vi "connection state machine.vi"(11 "connection in":refnum<class "connection maintainer.lvclass">) -> ()   [LabVIEW 2015, in "connection maintainer.lvclass"]
uses:
  connection maintainer.lvclass
  communicator/communicator.lvclass/communicator.ctl
  message/communicator message.lvclass/communicator message.ctl
  connection maintainer.lvclass/connection maintainer.ctl
  message/create message.vi
  message/communicator message.lvclass
  communicator/communicator.lvclass
panel:
  out "error IO":errorcluster
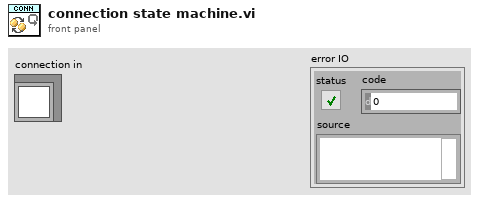
[diagram p1: front panel]
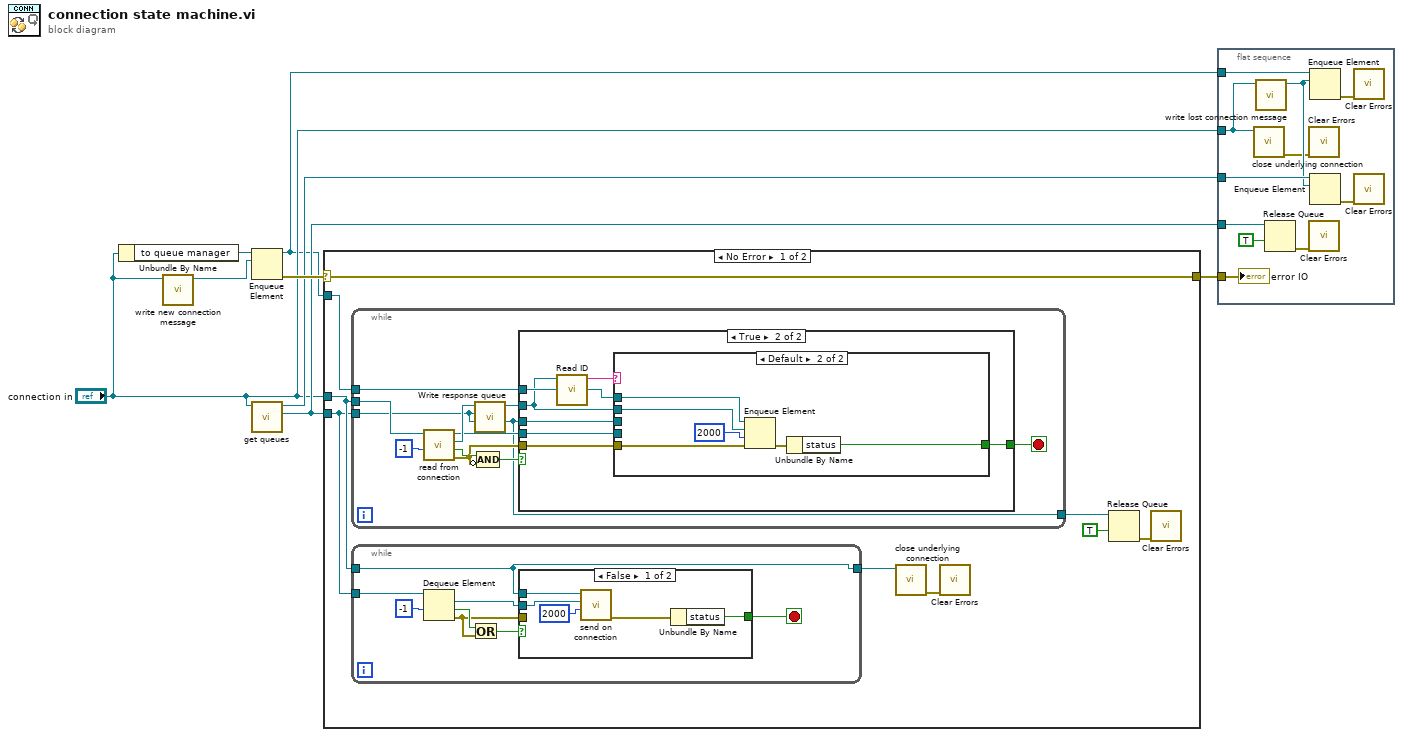
[diagram p0: block diagram]
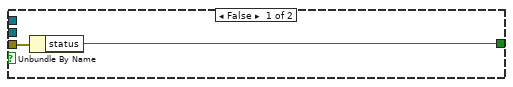
[diagram p2: hidden frame]
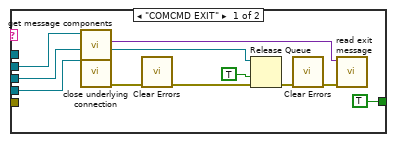
[diagram p3: hidden frame]
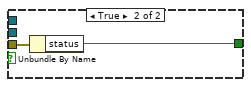
[diagram p4: hidden frame]
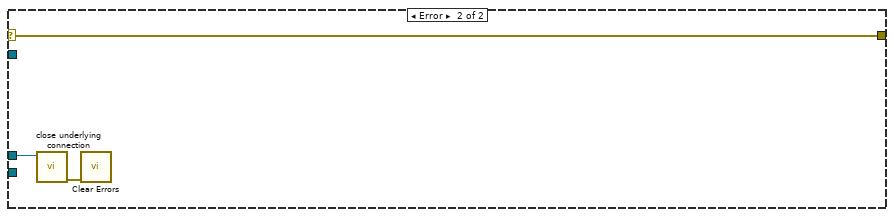
[diagram p5: hidden frame]
diagram:
  n1 = Unbundle By Name("connection in") -> ("to queue manager"=w3:refnum<queue>)
  n2 = call "write new connection message.vi"("connection"="connection in") -> ("element"=w8:refnum<class "communicator message.lvclass">)  [unwired: 10 in]
  n3 = Enqueue Element(queue=w3, element=w8) -> (queue out=w1:refnum<queue>, error out=w7:errorcluster)  [unwired: 2 in, 1 out]
  n4 = call "get queues.vi"("communicator in"="connection in") -> ("to worker"=w4:refnum<queue>, "to parent"=w5:refnum<queue>)  [unwired: 9 in]
  n5 = case shown="No Error" w7 {
    selector: w7 -> [w11 w69]
    tunnel: "connection in" -> [w17 w70]
    tunnel: w1 -> [w16 _]
    tunnel: w4 -> [w12 _]
    tunnel: [w11 w69] -> w6
    frame No Error {
      n6 = while {
        tunnel: w17 -> [w26]
        tunnel: w16 -> [w27]
        tunnel: [w18] -> w13
        tunnel: w12 -> [w18]
        stop <- w28 stop-if-true
        n7 = call-dynamic "read from connection.vi"("timeout ms (-1)"=-1 ("timeout ms (10000)"), "connection in"=w26) -> ("error out"=w22:errorcluster, "valid?"=w24:bool, "data message"=w20:refnum<class "communicator message.lvclass">, "connection out"=w19:refnum<class "connection maintainer.lvclass">)  [unwired: 6 in]
        n8 = call "Write response queue.vi"("response queue"=w18, "communicator message in"=w20) -> ("communicator message out"=w21:refnum<class "communicator message.lvclass">)  [unwired: 9 in]
        n9 = Compound Arithmetic op=AND(w24, invert w22) -> (w23:bool)
        n10 = case shown="True" w23 {
          tunnel: [w30 w36] -> w28
          tunnel: w27 -> [_ w37]
          tunnel: w21 -> [_ w34]
          tunnel: w22 -> [w29 w35]
          tunnel: w19 -> [_ w32]
          tunnel: w18 -> [_ w31]
          frame False {
            n11 = Unbundle By Name(w29) -> ("status"=w30:bool)
          }
          frame True {
            n12 = call "Read ID.vi"("communicator message in"=w34) -> ("ID"=w33:string)  [unwired: 10 in]
            n13 = case shown="Default" w33 {
              tunnel: w37 -> [_ w53]
              tunnel: [TRUE ("status") w50] -> w36
              tunnel: w34 -> [w46 w49]
              tunnel: w35 -> [_ w48]
              tunnel: w32 -> [w43 _]
              tunnel: w31 -> [w40 _]
              frame "COMCMD EXIT" {
                n14 = call "get message components.vi"("message"=w46) -> ("data"=w45:variant)  [unwired: 9 in, 1 out]
                n15 = call-dynamic "close underlying connection.vi"("connection in"=w43) -> ("error out"=w44:errorcluster)  [unwired: 10 in]
                n16 = call <vilib>:"Clear Errors.vi"("error in (no error)"=w44) -> ("error out"=w39:errorcluster)  [unwired: 5 in, 1 out]
                n17 = Release Queue(queue=w40, force destroy? (F)=TRUE, error in (no error)=w39) -> (error out=w42:errorcluster)  [unwired: 2 out]
                n18 = call <vilib>:"Clear Errors.vi"("error in (no error)"=w42) -> ("error out"=w38:errorcluster)  [unwired: 5 in, 1 out]
                n19 = call "read exit message.vi"("error in"=w38, "data"=w45) -> ()  [unwired: 9 in, 1 out]
              }
              frame Default {
                n20 = Enqueue Element(queue=w53, element=w49, timeout in ms (-1)=2000, error in (no error)=w48) -> (error out=w51:errorcluster)  [unwired: 2 out]
                n21 = Unbundle By Name(w51) -> ("status"=w50:bool)
              }
            }
          }
        }
      }
      n22 = while {
        tunnel: w12 -> [w61]
        tunnel: w17 -> [w54]
        tunnel: [w54] -> w10
        stop <- w57 stop-if-true
        n23 = Dequeue Element(queue=w61, timeout in ms (-1)=-1) -> (element=w55:refnum<class "communicator message.lvclass">, timed out?=w59:bool, error out=w58:errorcluster)  [unwired: 1 in, 1 out]
        n24 = Or(x=w59, y=w58) -> (x .or. y?=w56:bool)
        n25 = case shown="False" w56 {
          tunnel: w58 -> [_ w68]
          tunnel: [w66 w67] -> w57
          tunnel: w55 -> [w62 _]
          tunnel: w54 -> [w65 _]
          frame False {
            n26 = call-dynamic "send on connection.vi"("timeout ms (10000)"=2000, "data message"=w62, "connection in"=w65) -> ("error out"=w64:errorcluster)  [unwired: 7 in, 1 out]
            n27 = Unbundle By Name(w64) -> ("status"=w66:bool)
          }
          frame True {
            n28 = Unbundle By Name(w68) -> ("status"=w67:bool)
          }
        }
      }
      n29 = call-dynamic "close underlying connection.vi"("connection in"=w10) -> ("error out"=w9:errorcluster)  [unwired: 10 in]
      n30 = call <vilib>:"Clear Errors.vi"("error in (no error)"=w9) -> ()  [unwired: 5 in, 2 out]
      n31 = Release Queue(queue=w13, force destroy? (F)=TRUE) -> (error out=w14:errorcluster)  [unwired: 1 in, 2 out]
      n32 = call <vilib>:"Clear Errors.vi"("error in (no error)"=w14) -> ()  [unwired: 5 in, 2 out]
    }
    frame Error {
      n33 = call-dynamic "close underlying connection.vi"("connection in"=w70) -> ("error out"=w71:errorcluster)  [unwired: 10 in]
      n34 = call <vilib>:"Clear Errors.vi"("error in (no error)"=w71) -> ()  [unwired: 5 in, 2 out]
    }
  }
  n35 = flat-sequence {
    tunnel: w5 -> [w82]
    tunnel: "connection in" -> [w73]
    tunnel: w6 -> [w72]
    tunnel: w1 -> [w78]
    tunnel: w4 -> [w75]
    frame #0 {
      n36 = call-dynamic "close underlying connection.vi"("connection in"=w73) -> ("error out"=w74:errorcluster)  [unwired: 10 in]
      n37 = call "write lost connection message.vi"("connection"=w73) -> ("element"=w79:refnum<class "communicator message.lvclass">)  [unwired: 10 in]
      n38 = Release Queue(queue=w75, force destroy? (F)=TRUE) -> (error out=w77:errorcluster)  [unwired: 1 in, 2 out]
      n39 = call <vilib>:"Clear Errors.vi"("error in (no error)"=w74) -> ()  [unwired: 5 in, 2 out]
      n40 = call <vilib>:"Clear Errors.vi"("error in (no error)"=w77) -> ()  [unwired: 5 in, 2 out]
      n41 = Enqueue Element(queue=w78, element=w79) -> (error out=w80:errorcluster)  [unwired: 2 in, 2 out]
      n42 = Enqueue Element(queue=w82, element=w79) -> (error out=w81:errorcluster)  [unwired: 2 in, 2 out]
      n43 = call <vilib>:"Clear Errors.vi"("error in (no error)"=w80) -> ()  [unwired: 5 in, 2 out]
      n44 = call <vilib>:"Clear Errors.vi"("error in (no error)"=w81) -> ()  [unwired: 5 in, 2 out]
      "error IO" <- w72
    }
  }
